vi "send.status.vi"(6 "iteration":i32, 8 "error in (no error)":errorcluster, 11 "comic_crawler in":refnum<class "comic_crawler.lvclass">) -> (0 "error out":errorcluster, 2 "status":T1, 3 "comic_crawler out":refnum<class "comic_crawler.lvclass">)   [LabVIEW 2024, in "comic_crawler.lvclass"]
uses:
  comic_crawler.lvclass
  status--cluster.ctl
  comic_crawler.lvclass/comic_crawler.ctl
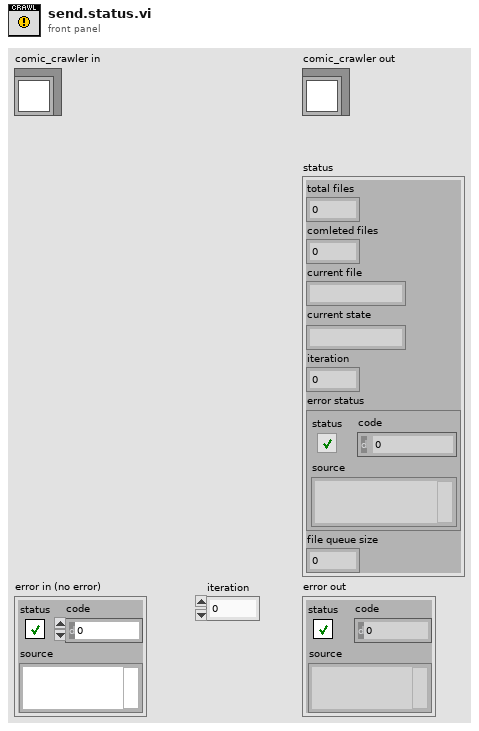
[diagram p1: front panel]
types:
  T1 = typedef "comic_crawler.lvclass/status--cluster.ctl" = cluster{"total files":i32, "comleted files":i32, "current file":string, "current state":string, "iteration":i32, "error status":errorcluster, "file queue size":i32}
  T2 = typedef "comic_crawler.lvclass/daemon.states--enum.ctl" = enum16{"start search", "idle", "set timer", "running", "stop search", "wait", "set delay", "shut down"}
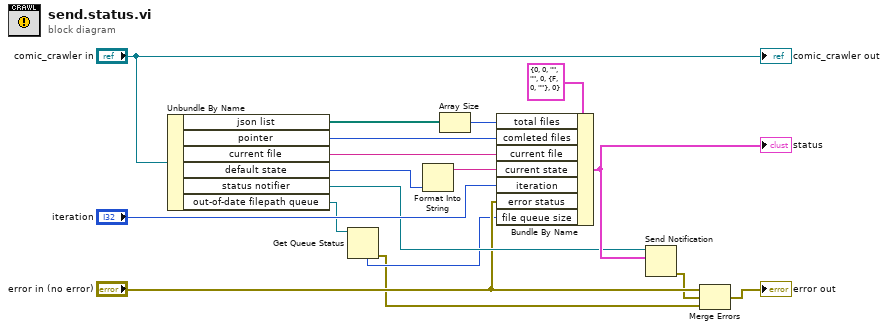
[diagram p0: block diagram]
diagram:
  n1 = Unbundle By Name("comic_crawler in") -> ("json list"=w13:path[], "pointer"=w11:i32, "current file"=w10:string, "default state"=w8:T2, "status notifier"=w7:refnum<notifier>, "out-of-date filepath queue"=w3:refnum<queue>)
  n2 = Get Queue Status(queue=w3) -> (error out=w1:errorcluster, # elements in queue=w2:i32)  [unwired: 2 in, 6 out]
  n3 = Format Into String(w8) -> (resulting string=w9:string)  [unwired: 3 in, 1 out]
  n4 = Array Size(array=w13) -> (size(s)=w12:i32)
  n5 = Bundle By Name(cluster=T1 {"total files"=0, "comleted files"=0, "current file"="", "current state"="", "iteration"=0, "error status"={"status"=FALSE, "code"=0, "source"=""}, "file queue size"=0} ("status"), "total files"=w12, "comleted files"=w11, "current file"=w10, "current state"=w9, "iteration"="iteration", "error status"="error in (no error)", "file queue size"=w2) -> (w16:T1)
  "status" <- w16
  n6 = Send Notification(notification=w16, notifier=w7) -> (error out=w5:errorcluster)  [unwired: 1 in, 1 out]
  n7 = Merge Errors("error in (no error)", w5, w1) -> (→"error out":errorcluster)
  "comic_crawler out" <- "comic_crawler in"
